vi "Start Receiving.vi"(8 "error in (no error)":errorcluster, 10 "Input":T1, 11 "Vision Receiver in":refnum<class "Vision Receiver.lvclass">) -> (0 "error out":errorcluster, 3 "Vision Receiver out":refnum<class "Vision Receiver.lvclass">)   [LabVIEW 2022 SP3, in "Vision.lvlib" / "Vision Receiver.lvlib" / "Vision Receiver.lvclass"]
uses:
  Vision Receiver.lvclass
  UDP Input.ctl
  Vision Receiver.lvclass/Vision Receiver.ctl
  UDP Reader/UDP Reader Messages/Request Msg/Request Msg.lvclass/Request Msg.ctl
  <vilib>/ActorFramework/Message Enqueuer/Message Enqueuer.lvclass/Message Enqueuer.ctl
  <vilib>/ActorFramework/Message Enqueuer/Enqueue.vi
  UDP Reader/UDP Reader Messages/Request Msg/Request Msg.lvclass
  C:/Program Files (x86)/National Instruments/LabVIEW 2022/vi.lib/ActorFramework/Message/Message.lvclass
  <vilib>/ActorFramework/Message Priority Queue/Priority Enqueue.vi
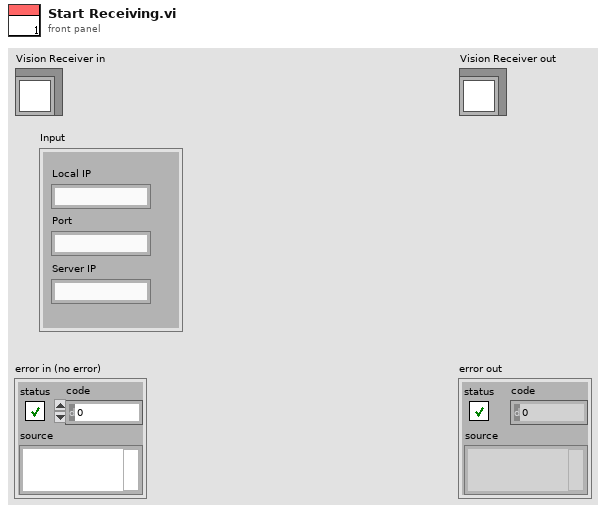
[diagram p1: front panel]
types:
  T1 = typedef "UDP Input.ctl" = cluster{"Local IP":string, "Port":string, "Server IP":string}
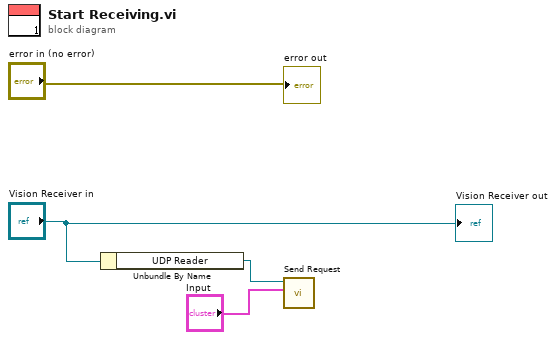
[diagram p0: block diagram]
diagram:
  n1 = Unbundle By Name("Vision Receiver in") -> ("UDP Reader"=w3:refnum<class "Message Enqueuer.lvclass">)
  n2 = call "Send Request.vi"("Input"="Input", "Message Enqueuer in"=w3) -> ()  [unwired: 8 in, 2 out]
  "error out" <- "error in (no error)"
  "Vision Receiver out" <- "Vision Receiver in"
